vi "4110_Current _Chan Config Dialog.vi"(8 "error in (no error)":errorcluster, 11 "Data Entry Limits:Maximum":dbl) -> (0 "error out":errorcluster, 1 "sense (out)":T1=1008 items=["Local"=1008, "Remote"=1009], 2 "Voltage Limit (out)":dbl, 3 "Initial Current Value (out)":dbl, 4 "Cancel (out)":bool, 5 "Number of Current Channels to Add? (out)":i16)   [LabVIEW 2015, in "NI PXI-4110 Programmable Power Supply Custom Device.lvlib"]
uses:
  NI PXI-4110 Programmable Power Supply Custom Device.lvlib
  <instrlib>/niDCPower/nidcpower.llb/niDCPower Sense.ctl
panel:
  in  "Cancel":bool
  in  "OK Button":bool
  in  "Voltage Limit":dbl format="%.4f"
  in  "Initial Current Value":dbl
  in  "sense":T1=1008 caption="Sense" items=["Local"=1008, "Remote"=1009]
  in  "Number of Current Channels to Add?":i16
  # "Current Channels"
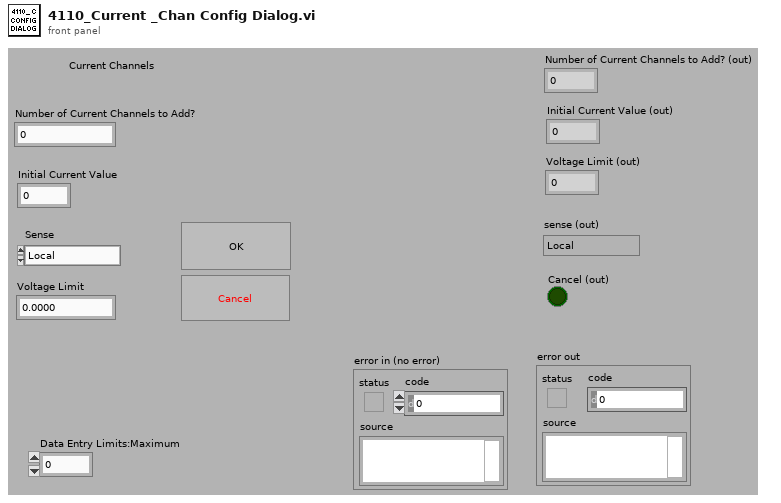
[diagram p1: front panel]
types:
  T1 = typedef "niDCPower Sense.ctl" = i32
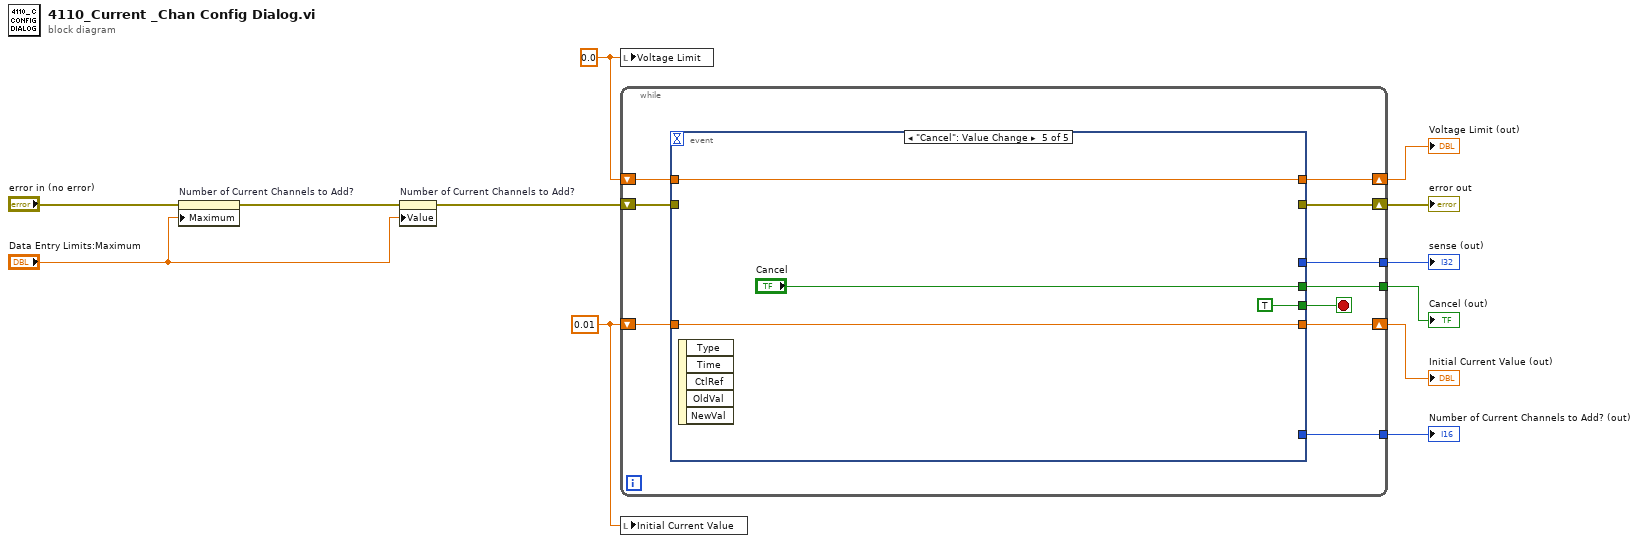
[diagram p0: block diagram]
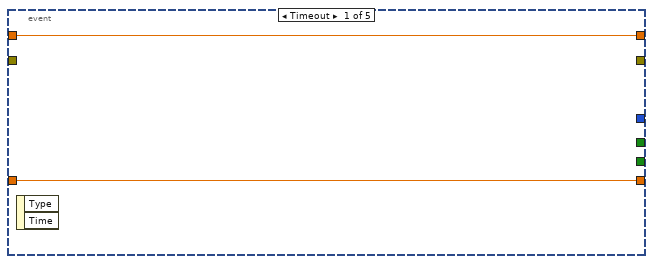
[diagram p2: hidden frame]
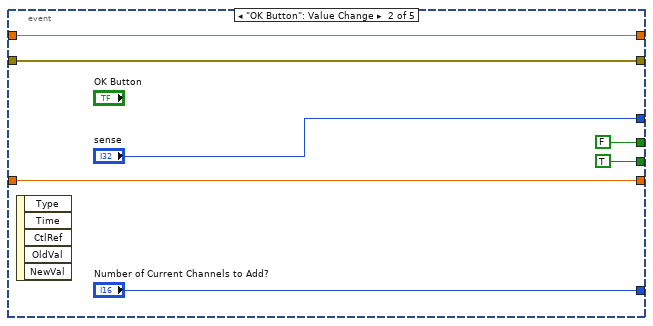
[diagram p3: hidden frame]
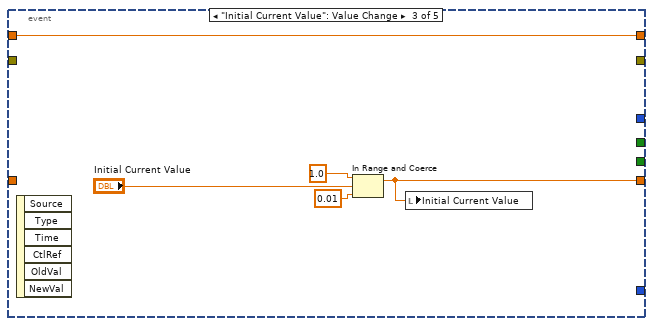
[diagram p4: hidden frame]
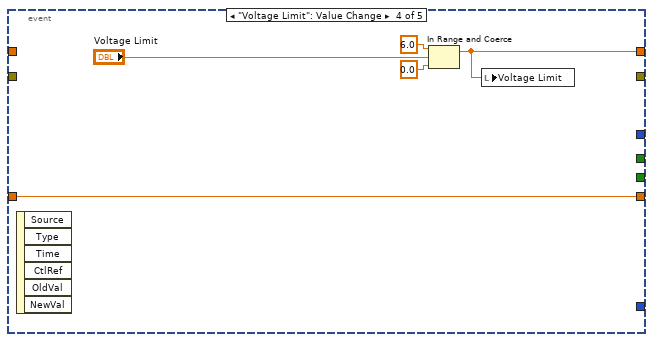
[diagram p5: hidden frame]
diagram:
  w2 = 0.0 ("Voltage Limit")
  w1 = 0.01 ("Initial Current Value")
  n1 = property on="Number of Current Channels to Add?" class="DigNum (strict)"(error in="error in (no error)", "Maximum"="Data Entry Limits:Maximum") -> (error out=w12:errorcluster)  [unwired: 1 in, 1 out]
  n2 = property on="Number of Current Channels to Add?" class="DigNum (strict)"(error in=w12, "Value"="Data Entry Limits:Maximum") -> (error out=w10:errorcluster)  [unwired: 1 in, 1 out]
  n3 = local write "Voltage Limit"(w2) -> ()
  n4 = while {
    tunnel: [w19] -> w7
    tunnel: [w17] -> w5
    tunnel: [w16] -> w3
    shift-right: [w21] -> w9
    shift-left: w10 -> [w22]
    shift-right: [w18] -> w6
    shift-left: w1 -> [w14]
    shift-right: [w20] -> w8
    shift-left: w2 -> [w13]
    stop <- w15 stop-if-true
    n5 = event shown="[4] \"Cancel\": Value Change" {
      selector: _ -> [_ _ _ _ _]
      dyn-events: _ -> [_ _ _ _ _]
      timeout: _ -> [_ _ _ _ _]
      tunnel: [w23 w25 w33 w39 w42] -> w20
      tunnel: [_ "sense" _ _ _] -> w19
      tunnel: [w24 w26 w32 w41 w43] -> w18
      tunnel: w22 -> [_ w30 _ _ _]
      tunnel: [_ w30 _ _ _] -> w21
      tunnel: [_ FALSE ("Cancel") _ _ "Cancel"] -> w17
      tunnel: [_ "Number of Current Channels to Add?" _ _ _] -> w16
      tunnel: [_ TRUE ("Cancel") _ _ TRUE ("Cancel")] -> w15
      tunnel: w14 -> [w24 w26 _ w41 w43]
      tunnel: w13 -> [w23 w25 w33 _ w42]
      event Timeout {
        n6 = event-data() -> ()  [unwired: 1 in, 2 out]
      }
      event "OK Button": Value Change {
        n7 = event-data() -> ()  [unwired: 1 in, 5 out]
      }
      event "Initial Current Value": Value Change {
        n8 = event-data() -> ()  [unwired: 1 in, 6 out]
        n9 = In Range and Coerce(upper limit=1.0, x="Initial Current Value", lower limit=0.01) -> (coerced(x)=w32:dbl)  [unwired: 1 out]
        n10 = local write "Initial Current Value"(w32) -> ()
      }
      event "Voltage Limit": Value Change {
        n11 = event-data() -> ()  [unwired: 1 in, 6 out]
        n12 = In Range and Coerce(upper limit=6.0, x="Voltage Limit", lower limit=0.0) -> (coerced(x)=w39:dbl)  [unwired: 1 out]
        n13 = local write "Voltage Limit"(w39) -> ()
      }
      event "Cancel": Value Change {
        n14 = event-data() -> ()  [unwired: 1 in, 5 out]
      }
    }
  }
  "error out" <- w9
  "Voltage Limit (out)" <- w8
  "sense (out)" <- w7
  "Initial Current Value (out)" <- w6
  "Cancel (out)" <- w5
  "Number of Current Channels to Add? (out)" <- w3
  n15 = local write "Initial Current Value"(w1) -> ()
